vi "LarCommand.vi"(0 "VISA in":refnum<visa-resource-name>="COM1", 1 "Parameter":i32, 4 "Command":T1(ring)) -> (6 "VISA out":refnum<visa-resource-name>, 7 "Answer":i32)   [LabVIEW 2009]
doc: "Envoie la Command et son Parameter au moteur connecté sur VISA in. \nSi la Command est SEL (selection du moteur), Parameter doit être le numero du moteur."
uses:
  <vilib>/Instr/_visa.llb/VISA Configure Serial Port (Serial Instr).vi
panel:
  out "read buffer":string
  out "error out":errorcluster
  in  "error in (no error)":errorcluster
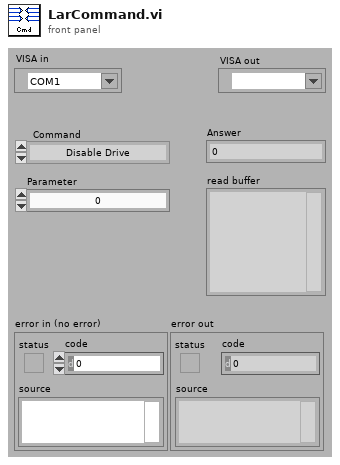
[diagram p1: front panel]
types:
  T1 = enum16{"Disable Drive", "Enable Drive", "Enable Program", "Get Actual Position", "Get Maximum Speed", "Get Acceleration", "Get Status", "Get Temperature", "Get Program Sequence", "Load Absolute Position", "Load Relative Position", "Load Maximum Speed", "Initiate Motion"}
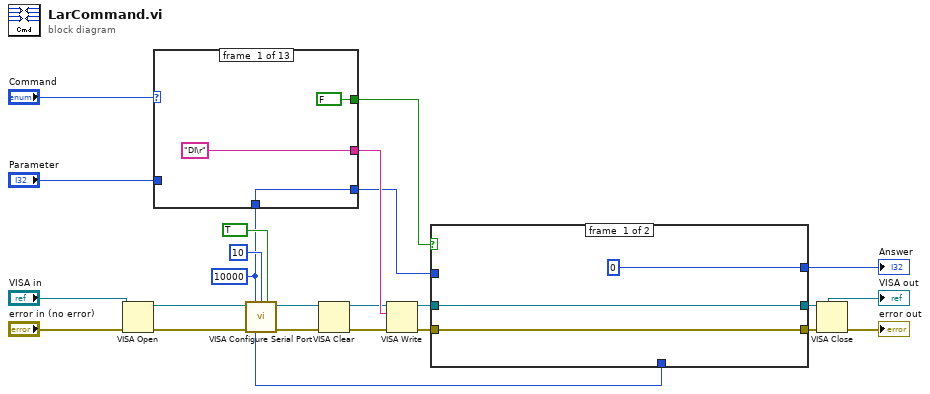
[diagram p0: block diagram]
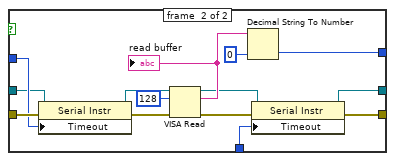
[diagram p2: hidden frame]
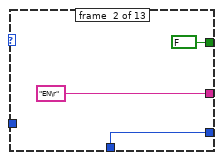
[diagram p3: hidden frame]
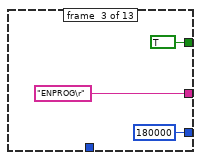
[diagram p4: hidden frame]
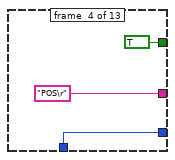
[diagram p5: hidden frame]
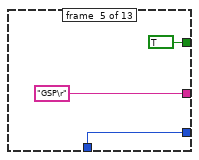
[diagram p6: hidden frame]
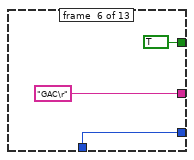
[diagram p7: hidden frame]
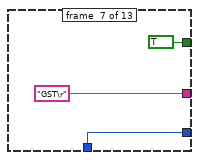
[diagram p8: hidden frame]
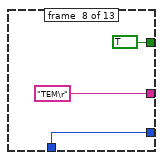
[diagram p9: hidden frame]
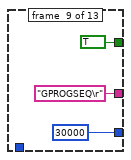
[diagram p10: hidden frame]
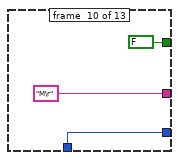
[diagram p11: hidden frame]
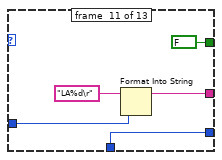
[diagram p12: hidden frame]
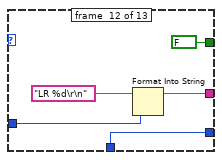
[diagram p13: hidden frame]
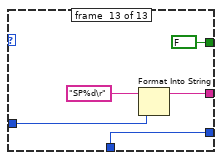
[diagram p14: hidden frame]
diagram:
  w1 = u32 10000 ("timeout (10sec)")
  n1 = VISA Open(error in (no error)="error in (no error)", VISA resource name="VISA in") -> (VISA resource name=w10:refnum<visa-resource-name>, error out=w12:errorcluster)  [unwired: 3 in]
  n2 = case shown="\"Enable Program\"" "Command" {
    tunnel: "Parameter" -> [_ _ _ _ _ _ _ _ _ _ w55 w60 w65]
    tunnel: ["DI\r" ("chaîne de format") "EN\r" ("chaîne de format") "ENPROG\r" ("chaîne de format") "POS\r" ("chaîne de format") "GSP\r" ("chaîne de format") "GAC\r" ("chaîne de format") "GST\r" ("chaîne de format") "TEM\r" ("chaîne de format") "GPROGSEQ\r" ("chaîne de format") "M\r" ("chaîne de format") w56 w61 w66] -> w20
    tunnel: [FALSE FALSE TRUE TRUE TRUE TRUE TRUE TRUE TRUE FALSE FALSE FALSE FALSE] -> w19
    tunnel: [w23 w26 u32 180000 ("timeout (10sec)") w32 w35 w38 w41 w44 u32 30000 ("General Settings:Timeout Value") w50 w53 w58 w63] -> w2
    tunnel: w1 -> [w23 w26 _ w32 w35 w38 w41 w44 _ w50 w53 w58 w63]
    frame #0 {
    }
    frame #1 {
    }
    frame #2 {
    }
    frame #3 {
    }
    frame #4 {
    }
    frame #5 {
    }
    frame #6 {
    }
    frame #7 {
    }
    frame #8 {
    }
    frame #9 {
    }
    frame #10 {
      n3 = Format Into String(format string="LA%d\r" ("chaîne de format"), w55) -> (resulting string=w56:string)  [unwired: 2 in, 1 out]
    }
    frame #11 {
      n4 = Format Into String(format string="LR %d\r\n" ("chaîne de format"), w60) -> (resulting string=w61:string)  [unwired: 2 in, 1 out]
    }
    frame #12 {
      n5 = Format Into String(format string="SP%d\r" ("chaîne de format"), w65) -> (resulting string=w66:string)  [unwired: 2 in, 1 out]
    }
  }
  n6 = call-poly "VISA Configure Serial Port"("VISA resource name"=w10, "timeout (10sec)"=w1, "termination char\n(0xA = '\\n' = LF)"=u8 10 ("termination char\n(0xA = '\\n' = LF)"), "Enable Termination\nChar (T)"=TRUE ("Enable Termination\nChar (T)"), "error in (no error)"=w12) -> ("VISA resource name out"=w9:refnum<visa-resource-name>, "error out"=w11:errorcluster)  [unwired: 9 in]
  n7 = VISA Clear(VISA resource name=w9, error in (no error)=w11) -> (VISA resource name out=w7:refnum<visa-resource-name>, error out=w8:errorcluster)
  n8 = VISA Write(VISA resource name=w7, write buffer=w20, error in (no error)=w8) -> (VISA resource name out=w4:refnum<visa-resource-name>, error out=w3:errorcluster)  [unwired: 1 out]
  n9 = case shown="True" w19 {
    tunnel: [w70 w73] -> w16
    tunnel: w3 -> [w70 w80]
    tunnel: [w69 w74] -> w14
    tunnel: w4 -> [w69 w77]
    tunnel: [0 ("default value 1") w81] -> w13
    tunnel: w2 -> [_ w78]
    tunnel: w1 -> [_ w71]
    frame #0 {
    }
    frame #1 {
      n10 = property class="Serial Instr"(reference=w77, error in=w80, "Timeout"=w78) -> (reference out=w76:refnum<visa-resource-name>, error out=w79:errorcluster)
      n11 = VISA Read(VISA resource name=w76, byte count=u32 128, error in (no error)=w79) -> (VISA resource name out=w75:refnum<visa-resource-name>, read buffer=w83:string, error out=w72:errorcluster)  [unwired: 1 out]
      "read buffer" <- w83
      n12 = Decimal String To Number(string=w83, default (0L)=0 ("default value 1")) -> (number=w81:i32)  [unwired: 1 in, 1 out]
      n13 = property class="Serial Instr"(reference=w75, error in=w72, "Timeout"=w71) -> (reference out=w74:refnum<visa-resource-name>, error out=w73:errorcluster)
    }
  }
  "Answer" <- w13
  "VISA out" <- w14
  n14 = VISA Close(VISA resource name=w14, error in (no error)=w16) -> (error out=→"error out":errorcluster)
